vi "Read Modbus Settings.vi"(11 "appended path":path) -> (0 "error out":errorcluster, 3 "Ini File":T1(array[cluster]))   [LabVIEW 2021]
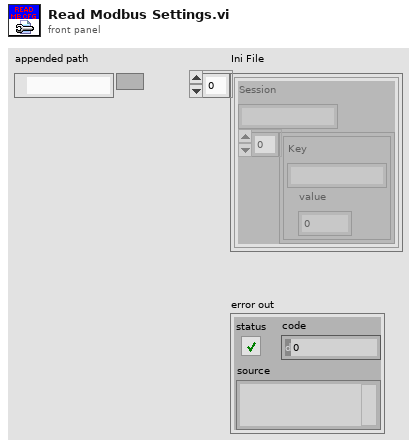
[diagram p1: front panel]
types:
  T1 = cluster{"Session":string, cluster{"Key":string, "value":u32}[]}[]
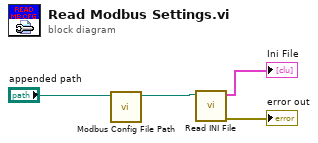
[diagram p0: block diagram]
diagram:
  n1 = call "Modbus Config File Path.vi"("appended path in"="appended path") -> ("appended path out"=w3:path)  [unwired: 10 in]
  n2 = call "Read INI File.vi"("name or relative path"=w3) -> ("error out"=→"error out":errorcluster, "Ini File"=→"Ini File":T1)  [unwired: 9 in]
